vi "PID Get Error.vi"(4 "setpoint low":dbl, 6 "setpoint high":dbl, 7 "linearity":dbl, 9 "process variable":dbl, 10 "beta":dbl, 11 "setpoint":dbl) -> (1 "non-linear integral action":dbl, 2 "error with beta":dbl, 3 "error":dbl)   [LabVIEW 2017, in "NI_FunctionBlock Libraries.lvlib"]
uses:
  <vilib>/functionblocks/NI_FunctionBlock Libraries.lvlib
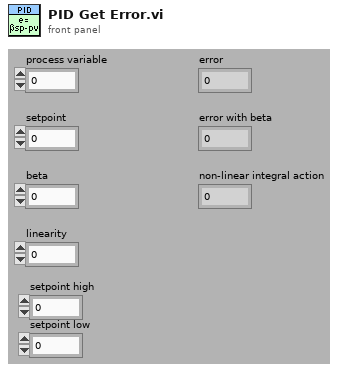
[diagram p1: front panel]
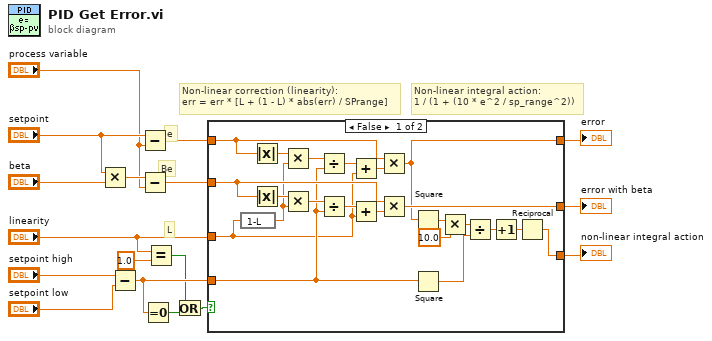
[diagram p0: block diagram]
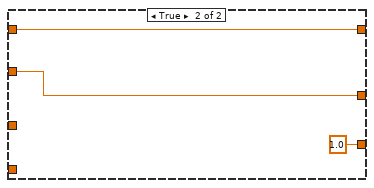
[diagram p2: hidden frame]
diagram:
  # "Non-linear correction (linearity):\nerr = err * [L + (1 - L) * abs(err) / SPrange]"
  # "Non-linear integral action:\n1 / (1 + (10 * e^2 / sp_range^2))"
  # "Be"
  # "e"
  # "L"
  n1 = Multiply(x="setpoint", y="beta") -> (x*y=w14:dbl)
  n2 = Subtract(x="setpoint high", y="setpoint low") -> (x-y=w17:dbl)
  n3 = Subtract(x="setpoint", y="process variable") -> (x-y=w15:dbl)
  n4 = Subtract(x=w14, y="process variable") -> (x-y=w16:dbl)
  n5 = Equal To 0?(x=w17) -> (x = 0?=w3:bool)
  n6 = Equal?(x="linearity", y=1.0) -> (x = y?=w4:bool)
  n7 = Or(x=w4, y=w3) -> (x .or. y?=w5:bool)
  n8 = case shown="False" w5 {
    tunnel: [w25 1.0 ("t")] -> w9
    tunnel: w15 -> [w30 w41]
    tunnel: w16 -> [w31 w40]
    tunnel: [w21 w41] -> w10
    tunnel: [w29 w40] -> w11
    tunnel: w17 -> [w26 _]
    tunnel: "linearity" -> [w24 _]
    frame False {
      n9 = expression code="1-L"(w24) -> (w23:dbl)
      n10 = Absolute Value(x=w30) -> (abs(x)=w39:dbl)
      n11 = Absolute Value(x=w31) -> (abs(x)=w32:dbl)
      n12 = Multiply(x=w39, y=w23) -> (x*y=w38:dbl)
      n13 = Multiply(x=w32, y=w23) -> (x*y=w33:dbl)
      n14 = Divide(x=w38, y=w26) -> (x/y=w37:dbl)
      n15 = Divide(x=w33, y=w26) -> (x/y=w34:dbl)
      n16 = Add(x=w37, y=w24) -> (x+y=w36:dbl)
      n17 = Add(x=w34, y=w24) -> (x+y=w35:dbl)
      n18 = Multiply(x=w30, y=w36) -> (x*y=w21:dbl)
      n19 = Multiply(x=w31, y=w35) -> (x*y=w29:dbl)
      n20 = Square(x=w21) -> (x^2=w19:dbl)
      n21 = Square(x=w26) -> (x^2=w28:dbl)
      n22 = Multiply(x=w19, y=10.0) -> (x*y=w18:dbl)
      n23 = Divide(x=w18, y=w28) -> (x/y=w22:dbl)
      n24 = Increment(x=w22) -> (x+1=w27:dbl)
      n25 = Reciprocal(x=w27) -> (1/x=w25:dbl)
    }
    frame True {
    }
  }
  "error with beta" <- w11
  "error" <- w10
  "non-linear integral action" <- w9
